vi "Image Correction.vi"() -> ()   [LabVIEW 2014]
uses:
  <vilib>/vision/Calibration.llb/Distortion Model.ctl
  <vilib>/vision/Calibration.llb/Distortion Model Types.ctl
  <vilib>/vision/NI_Vision_Development_Module.lvlib
panel:
  out "Src":T1(plugin-control)
  out "Corrected":T1(plugin-control)
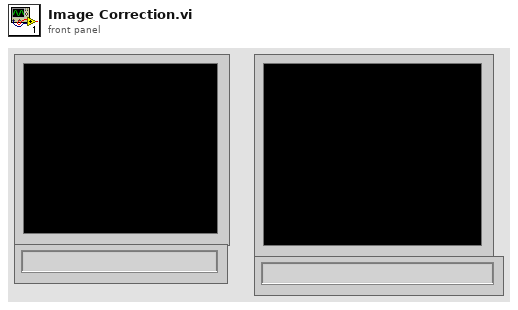
[diagram p1: front panel]
types:
  T1 = typedef "IMAQ Image.ctl" = refnum<image>
  T2 = cluster{"Corrected Image Scaling":u32, "Corrected Image Learn ROI":u32, "Learn Correction Table?":bool}
  T3 = typedef "Distortion Model.ctl" = cluster{"Distortion Model":T4, "Polynomial Model Setup":cluster{"Radial Coefficient":u32, "Tangential Coefficients ":bool}}
  T4 = typedef "Distortion Model Types.ctl" = i32
  T5 = typedef "Image Unit" = enum32{"Undefined", "Angström", "Micrometer", "Millimeter", "Centimeter", "Meter", "Kilometer", "Microinch", "Inch", "Feet", "Nautical miles", "Standard miles", "Steps"}
  T6 = typedef "Calibration Reference Points.ctl" = cluster{"Pixel Coordinates":cluster{"X":dbl, "Y":dbl}[], "Real World Coordinates":cluster{"X":dbl, "Y":dbl}[], "Unit":T5, "Image Size":cluster{"X":u32, "Y":u32}}
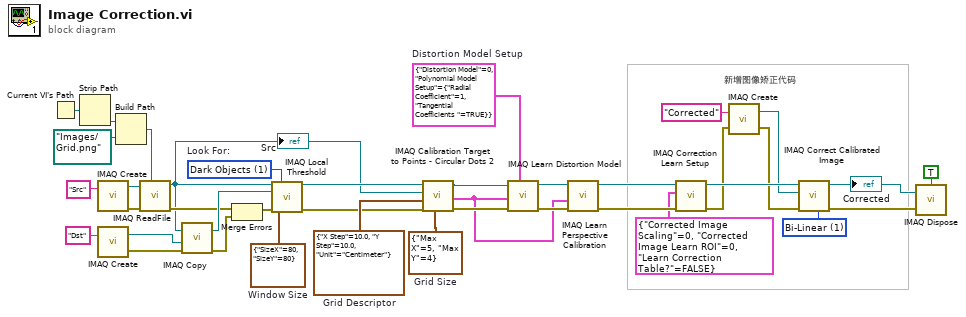
[diagram p0: block diagram]
diagram:
  w6 = u32 1 items=["Zero Order", "Bi-Linear", "Quadratic", "Cubic Spline"] ("Interpolation Type")
  w27 = T3 {"Distortion Model"=0, "Polynomial Model Setup"={"Radial Coefficient"=1, "Tangential Coefficients "=TRUE}}  # Distortion Model Setup
  w28 = cluster{"SizeX":i32, "SizeY":i32} {"SizeX"=80, "SizeY"=80}  # Window Size
  w29 = u32 1 items=["Bright Objects", "Dark Objects"]  # Look For:
  w30 = cluster{"Max X":u32, "Max Y":u32} {"Max X"=5, "Max Y"=4}  # Grid Size
  w32 = cluster{"X Step":sgl, "Y Step":sgl, "Unit":T5} {"X Step"=10.0, "Y Step"=10.0, "Unit"=enum."Centimeter"}  # Grid Descriptor
  # "新增图像矫正代码"
  n1 = Current VI's Path() -> (path=w35:path)
  n2 = Strip Path(path=w35) -> (stripped path=w34:path)  [unwired: 1 out]
  n3 = call "IMAQ Create"("Image Name"="Src") -> ("New Image"=w39:T1, "error out"=w38:errorcluster)  [unwired: 4 in]
  n4 = call "IMAQ Create"("Image Name"="Dst") -> ("New Image"=w20:T1, "error out"=w21:errorcluster)  [unwired: 4 in]
  n5 = Build Path(base path=w34, name or relative path=path "Images/Grid.png" ("prompt")) -> (appended path=w33:path)
  n6 = call "IMAQ ReadFile"("File Path"=w33, "error in (no error)"=w38, "Image"=w39) -> ("error out"=w17:errorcluster, "Image Out"=w13:T1)  [unwired: 4 in, 3 out]
  "Src" <- w13
  n7 = call "IMAQ Copy"("error in (no error)"=w21, "Image Dst"=w20, "Image Src"=w13) -> ("error out"=w16:errorcluster, "Image Dst Out"=w19:T1)  [unwired: 3 in]
  n8 = Merge Errors(w17, w16) -> (w15:errorcluster)
  n9 = call "IMAQ Local Threshold"("Image Src"=w13, "Look For (Bright Objects)"=w29, "Image Dst"=w19, "Window Size (32x32)"=w28, "error in (no error)"=w15) -> ("Image Dst Out"=w18:T1, "error out"=w25:errorcluster)  [unwired: 9 in]
  n10 = call "IMAQ Calibration Target to Points - Circular Dots 2"("Grid Size"=w30, "error in (no error)"=w25, "Grid Descriptor"=w32, "Grayscale Image"=w13, "Target Image"=w18) -> ("error out"=w24:errorcluster, "Reference Points"=w23:T6, "Target Image (dup)"=w12:T1)  [unwired: 4 in]
  n11 = call "IMAQ Learn Distortion Model"("Distortion Model Setup"=w27, "error in (no error)"=w24, "Reference Points"=w23, "Calibration Template Image"=w12) -> ("error out"=w26:errorcluster, "Calibration Template Image Out"=w14:T1)  [unwired: 2 in, 4 out]
  n12 = call "IMAQ Learn Perspective Calibration"("error in (no error)"=w26, "Reference Points"=w23, "Calibration Template Image"=w14) -> ("error out"=w11:errorcluster, "Calibration Template Image Out"=w10:T1)  [unwired: 1 in, 6 out]
  n13 = call "IMAQ Correction Learn Setup"("error in (no error)"=w11, "Correction Learn Setup"=T2 {"Corrected Image Scaling"=0, "Corrected Image Learn ROI"=0, "Learn Correction Table?"=FALSE}, "Calibration Template Image"=w10) -> ("error out"=w3:errorcluster, "Calibration Template Image Out"=w9:T1)  [unwired: 7 in]
  n14 = call "IMAQ Create"("Image Name"="Corrected", "error in (no error)"=w3) -> ("New Image"=w1:T1, "error out"=w2:errorcluster)  [unwired: 3 in]
  n15 = call "IMAQ Correct Calibrated Image"("Interpolation Type"=w6, "error in (no error)"=w2, "Image Dst"=w1, "Image Src"=w9) -> ("error out"=w8:errorcluster, "Corrected Image"=w5:T1)  [unwired: 6 in]
  "Corrected" <- w5
  n16 = call "IMAQ Dispose"("All Images? (No)"=TRUE, "Image"=w5, "error in (no error)"=w8) -> ()  [unwired: 3 in, 1 out]
